vi "Weather Station UI.vi"() -> ()   [LabVIEW 2019]
uses:
  Supporting Files/Weather Station States.ctl
  Supporting Files/Weather Data.ctl
  <vilib>/DAQmx/read.llb/DAQmx Read (Analog DBL 1Chan 1Samp).vi
  <vilib>/DAQmx/create/channels.llb/DAQmx Create Channel (AI-Temperature-Thermocouple).vi
  <vilib>/DAQmx/miscellaneous.llb/DAQmx Fill In Error Info.vi
panel:
  in  "Stop":bool
  in  "Thermocouple Channel":tag="PCI-6221/ai0"
  out "Warning":string
  out "Temperature History":dbl(graph)
  in  "Lower Limit":dbl=20.0
  in  "Upper Limit":dbl=30.0
  # "Temperature Ranges (deg C)"
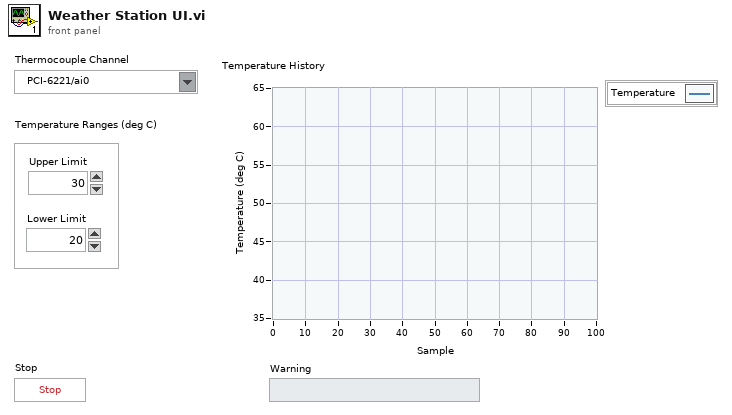
[diagram p1: front panel]
types:
  T1 = typedef "Weather Data.ctl" = cluster{"Current Temperature":dbl, "Max Temperature":dbl, "Min Temperature":dbl, "Warning?":bool, "Warning Text":string}
  T2 = typedef "Weather Station States.ctl" = enum16{"Initialize", "Acquire", "Analyze", "Log", "Check Time", "Shutdown"}
  T3 = enum16{"open", "replace", "create", "open or create", "replace or create", "replace or create with confirmation"}
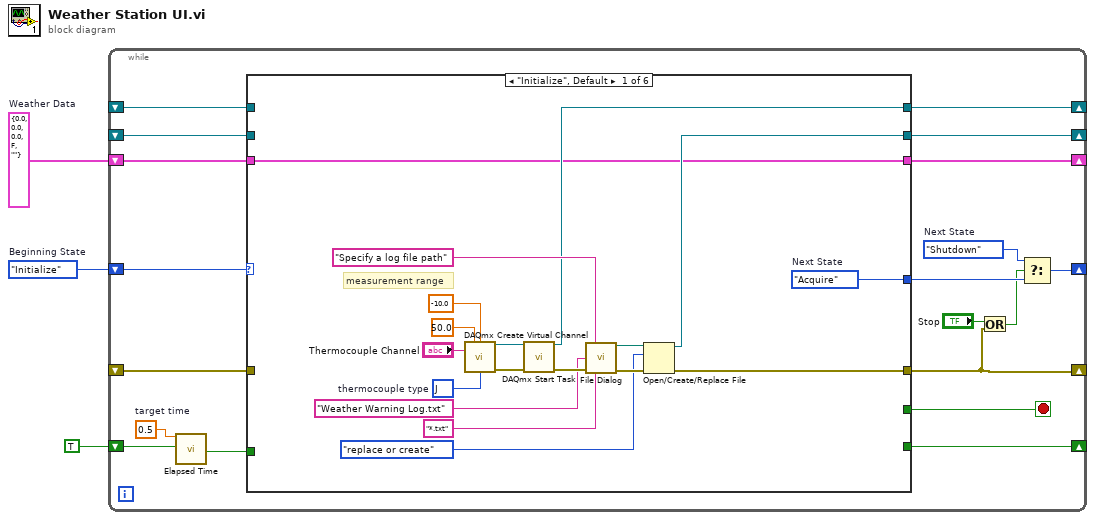
[diagram p0: block diagram]
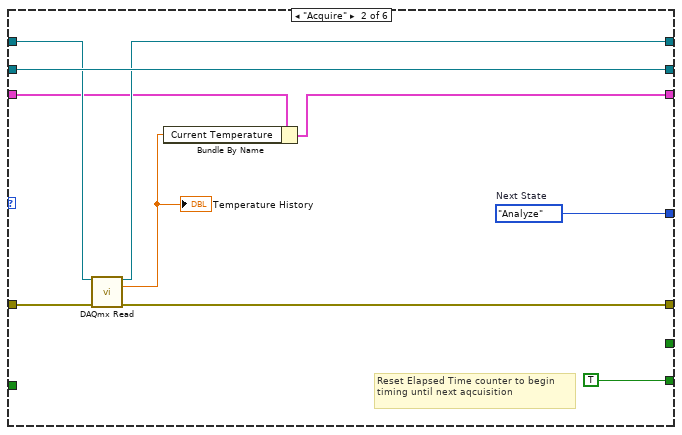
[diagram p2: hidden frame]
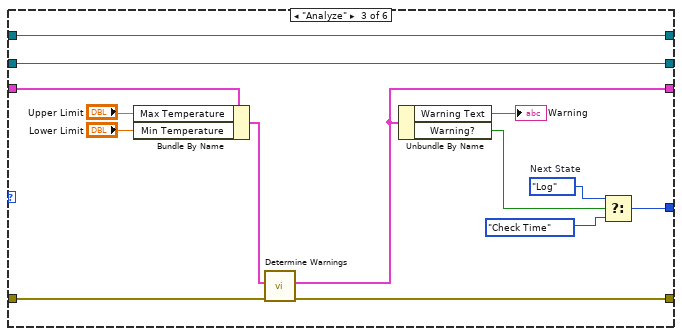
[diagram p3: hidden frame]
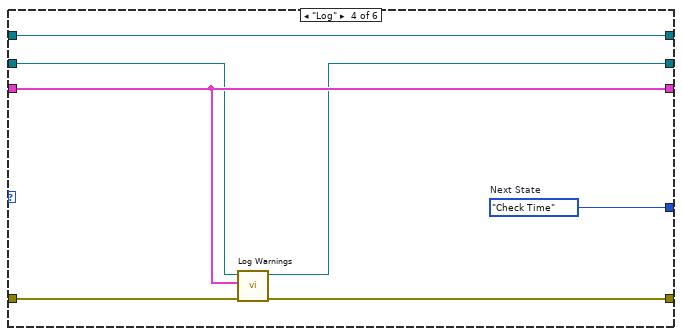
[diagram p4: hidden frame]
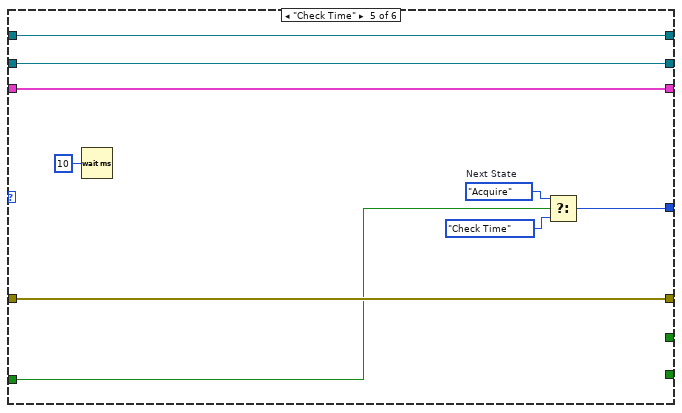
[diagram p5: hidden frame]
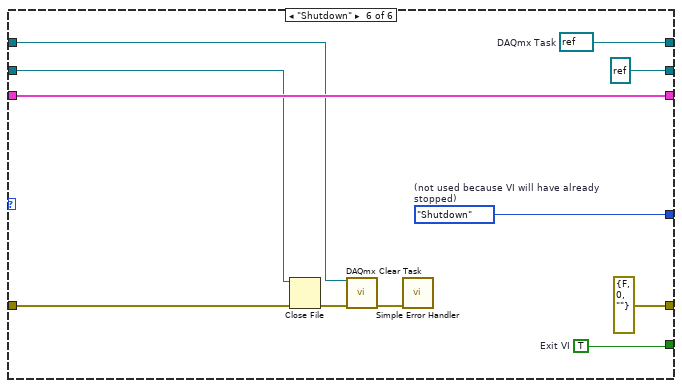
[diagram p6: hidden frame]
diagram:
  w2 = T1 {"Current Temperature"=0.0, "Max Temperature"=0.0, "Min Temperature"=0.0, "Warning?"=FALSE, "Warning Text"=""}  # Weather Data
  w3 = Weather_Station_States."Initialize"  # Beginning State
  n1 = while {
    shift-right: [w13] -> _
    shift-left: TRUE -> [w11]
    shift-right: [w15] -> _
    shift-left: w2 -> [w18]
    shift-right: [w8] -> _
    shift-left: w3 -> [w19]
    shift-right: [w16] -> _
    shift-left: _ -> [w21]
    shift-right: [w14] -> _
    shift-left: _ -> [w20]
    shift-right: [w6] -> _
    shift-left: _ -> [w17]
    stop <- w4 stop-if-true
    w10 = Weather_Station_States."Shutdown"  # Next State
    w22 = 0.5  # target time
    n2 = call "Elapsed Time"("Time Target (s)"=w22, "Reset"=w11) -> ("Time has Elapsed"=w12:bool)  [unwired: 10 in, 7 out]
    n3 = case shown="\"Initialize\", Default" w19 {
      tunnel: w21 -> [_ w47 w57 w71 w79 w82]
      tunnel: w20 -> [_ w50 w56 w67 w78 w83]
      tunnel: w18 -> [w25 w45 w64 w68 w77 w86]
      tunnel: w17 -> [_ w49 w63 w70 w76 w89]
      tunnel: [w25 w44 w60 w68 w77 w86] -> w15
      tunnel: [w26 w50 w56 w66 w78 refnum<file> refnum ("file ref out")] -> w14
      tunnel: [w23 w48 w62 w69 w76 errorcluster {"status"=FALSE, "code"=0, "source"=""} ("error constant")] -> w6
      tunnel: [w27 w46 w57 w71 w79 w85] -> w16
      tunnel: [w24 w41 w59 w65 w74 w81] -> w9
      tunnel: [_ TRUE _ _ _ _] -> w13
      tunnel: w12 -> [_ _ _ _ w75 _]
      tunnel: [_ _ _ _ _ w87] -> w4
      frame "Initialize", Default {
        w24 = Weather_Station_States."Acquire"  # Next State
        w38 = 10072 items=["J"=10072, "K"=10073, "N"=10077, "R"=10082, "S"=10085, "T"=10086, "B"=10047, "E"=10055]  # thermocouple type
        # "measurement range"
        n4 = call-poly <vilib>:"DAQmx Create Virtual Channel.vi"("maximum value"=50.0, "minimum value"=-10.0, "physical channels"="Thermocouple Channel", "thermocouple type"=w38) -> ("task out"=w37:refnum<k21>, "error out"=w36:errorcluster)  [unwired: 10 in]
        n5 = call <vilib>:"DAQmx Start Task.vi"("task/channels in"=w37, "error in"=w36) -> ("task out"=w27:refnum<k21>, "error out"=w33:errorcluster)  [unwired: 12 in]
        n6 = call "File Dialog"("prompt"="Specify a log file path", "default name"="Weather Warning Log.txt", "error in"=w33, "pattern (all files)"="*.txt") -> ("selected path"=w34:path, "error out"=w35:errorcluster)  [unwired: 8 in, 2 out]
        n7 = Open/Create/Replace File(file path (use dialog)=w34, error in=w35, operation (0:open)=T3."replace or create") -> (refnum out=w26:refnum<file>, error out=w23:errorcluster)  [unwired: 3 in, 1 out]
      }
      frame "Acquire" {
        w41 = Weather_Station_States."Analyze"  # Next State
        # "Reset Elapsed Time counter to begin timing until next aqcuisition"
        n8 = call-poly <vilib>:"DAQmx Read.vi"("task/channels in"=w47, "error in"=w49) -> ("task out"=w46:refnum<k21>, "data"=w42:dbl, "error out"=w48:errorcluster)  [unwired: 11 in]
        "Temperature History" <- w42
        n9 = Bundle By Name(cluster=w45, "Current Temperature"=w42) -> (w44:T1)
      }
      frame "Analyze" {
        w52 = Weather_Station_States."Log"  # Next State
        n10 = Bundle By Name(cluster=w64, "Max Temperature"="Upper Limit", "Min Temperature"="Lower Limit") -> (w61:T1)
        n11 = call "Determine Warnings.vi"("Error In"=w63, "Weather Data In"=w61) -> ("Error Out"=w62:errorcluster, "Weather Data Out"=w60:T1)  [unwired: 8 in]
        n12 = Unbundle By Name(w60) -> ("Warning Text"=→"Warning":string, "Warning?"=w58:bool)
        n13 = Select(t=w52, s=w58, f=Weather_Station_States."Check Time") -> (s? t:f=w59:T2)
      }
      frame "Log" {
        w65 = Weather_Station_States."Check Time"  # Next State
        n14 = call "Log Warnings.vi"("Error In"=w70, "Weather Data In"=w68, "file ref in"=w67) -> ("Error Out"=w69:errorcluster, "file ref out"=w66:refnum<file>)  [unwired: 7 in]
      }
      frame "Check Time" {
        w73 = Weather_Station_States."Acquire"  # Next State
        n15 = Wait (ms)(milliseconds to wait=u32 10) -> ()  [unwired: 1 out]
        n16 = Select(t=w73, s=w75, f=Weather_Station_States."Check Time") -> (s? t:f=w74:T2)
      }
      frame "Shutdown" {
        w81 = Weather_Station_States."Shutdown"  # (not used because VI will have already stopped)
        w85 = refnum<k21> refnum  # DAQmx Task
        w87 = TRUE  # Exit VI
        n17 = Close File(refnum=w83, error in=w89) -> (error out=w90:errorcluster)  [unwired: 1 out]
        n18 = call <vilib>:"DAQmx Clear Task.vi"("task in"=w82, "error in"=w90) -> ("error out"=w91:errorcluster)  [unwired: 13 in]
        n19 = call <vilib>:"Simple Error Handler.vi"("error in (no error)"=w91) -> ()  [unwired: 4 in, 5 out]
      }
    }
    n20 = Or(x="Stop", y=w6) -> (x .or. y?=w5:bool)
    n21 = Select(t=w10, s=w5, f=w9) -> (s? t:f=w8:T2)
  }
